vi "ProcessUDPValues.vi"(8 "error in (no error)":errorcluster, 11 "connection ID":refnum<k16>) -> ()   [LabVIEW 2015]
uses:
  GlobalVisionVars.vi
  navx-mxp/labview/navX Library v2/navX Library v2.lvlib
panel:
  out "ProcessTime":dbl
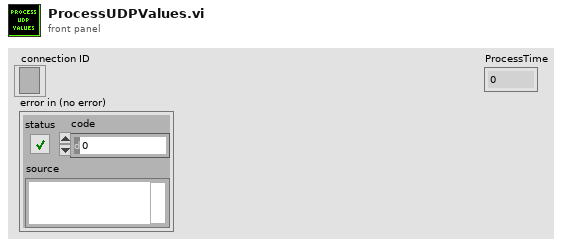
[diagram p1: front panel]
types:
  T1 = typedef "navX Library v2.lvlib/Z900_navX_DeviceTypeDef.ctl" = cluster{"Interface":cluster{"Protocol":T2, "Update Rate (4Hz-100Hz)":u8, "navX Open TypeDef":variant}, "Notify Packet":refnum<notifier>, "Loop VI Refnum":refnum<vi>, "Ready to Close Occurrence Refnum":refnum<k4>}
  T2 = typedef "navX Library v2.lvlib/Z900_navX_ProtocolTypeDef.ctl" = enum16{"SERIAL", "I2C", "SPI"}
  T3 = cluster{"Yaw":dbl, "Roll":dbl, "Pitch":dbl, "Heading":dbl, "Fused Heading":dbl}
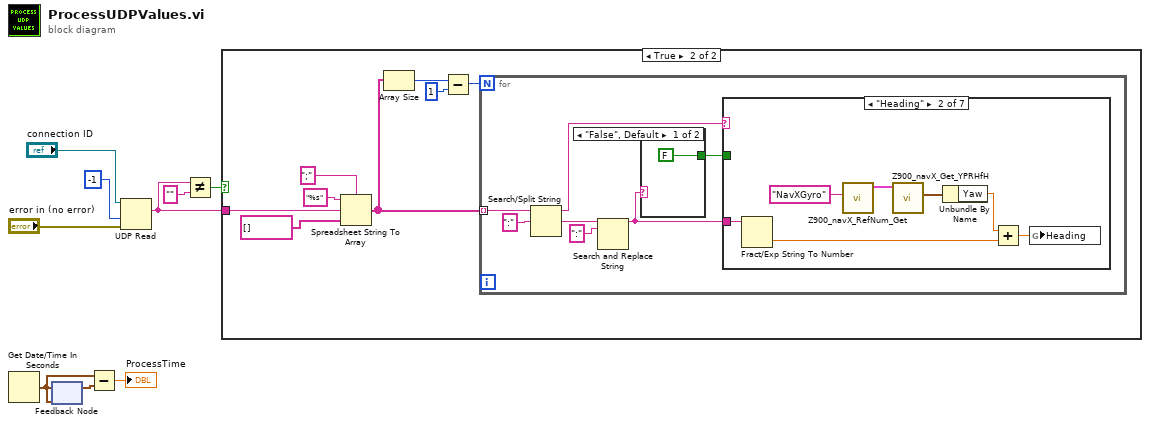
[diagram p0: block diagram]
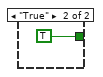
[diagram p3: hidden frame]
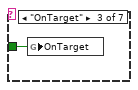
[diagram p5: hidden frame]
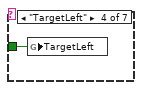
[diagram p6: hidden frame]
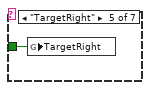
[diagram p7: hidden frame]
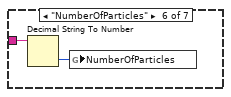
[diagram p8: hidden frame]
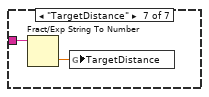
[diagram p9: hidden frame]
diagram:
  n1 = Get Date/Time In Seconds() -> (seconds since 1Jan1904=w7:timestamp)
  n2 = feedback-in #1(w7) -> ()
  n3 = feedback #1(w7) -> (w9:timestamp)
  n4 = Subtract(x=w7, y=w9) -> (x-y=→"ProcessTime":dbl)
  n5 = UDP Read(connection ID="connection ID", timeout ms (25000)=-1, 8:"error in (no error)") -> (data out=w1:string)  [unwired: 1 in, 4 out]
  n6 = Not Equal?(x=w1, y="") -> (x != y?=w2:bool)
  n7 = case shown="True" w2 {
    tunnel: w1 -> [_ w17]
    frame False {
    }
    frame True {
      n8 = Spreadsheet String To Array(delimiter (Tab)=";" ("search string/char (-)"), format string="%s", spreadsheet string=w17, array type (2D Dbl)=string[] []) -> (array=w13:string[])
      n9 = Array Size(array=w13) -> (size(s)=w12:i32)
      n10 = Subtract(x=w12, y=1) -> (x-y=w10:i32)
      n11 = for {
        N: w10 -> [_]
        tunnel: w13 -> [w24] mode=indexing
        n12 = Search/Split String(string=w24, search string/char (-)=":") -> (substring before match=w22:string, match + rest of string=w21:string)  [unwired: 1 in, 1 out]
        n13 = Search and Replace String(input string=w21, search string=":" ("replace string (\"\")")) -> (result string=w19:string)  [unwired: 6 in, 3 out]
        n14 = case shown="\"False\", Default" w19 {
          tunnel: [FALSE TRUE] -> w18
          frame "False", Default {
          }
          frame "True" {
          }
        }
        n15 = case shown="\"Heading\"" w22 {
          tunnel: w19 -> [_ w33 _ _ _ w38 w39]
          tunnel: w18 -> [_ _ w34 w35 w36 _ _]
          frame "False", Default {
          }
          frame "Heading" {
            n16 = Fract/Exp String To Number(string=w33) -> (number=w27:dbl)  [unwired: 3 in, 1 out]
            n17 = call "Z900_navX_RefNum_Get.vi"("refnum name"="NavXGyro") -> ("navX Device"=w32:T1)  [unwired: 9 in, 1 out]
            n18 = call "Z900_navX_Get_YPRHfH.vi"("navX Device"=w32) -> ("YRPHfH"=w31:T3)  [unwired: 7 in, 3 out]
            n19 = Unbundle By Name(w31) -> ("Yaw"=w29:dbl)
            n20 = Add(x=w29, y=w27) -> (x+y=w28:dbl)
            n21 = global write "GlobalVisionVars.vi" "Heading"(w28) -> ()
          }
          frame "OnTarget" {
            n22 = global write "GlobalVisionVars.vi" "OnTarget"(w34) -> ()
          }
          frame "TargetLeft" {
            n23 = global write "GlobalVisionVars.vi" "TargetLeft"(w35) -> ()
          }
          frame "TargetRight" {
            n24 = global write "GlobalVisionVars.vi" "TargetRight"(w36) -> ()
          }
          frame "NumberOfParticles" {
            n25 = Decimal String To Number(string=w38) -> (number=w37:i32)  [unwired: 2 in, 1 out]
            n26 = global write "GlobalVisionVars.vi" "NumberOfParticles"(w37) -> ()
          }
          frame "TargetDistance" {
            n27 = Fract/Exp String To Number(string=w39) -> (number=w40:dbl)  [unwired: 3 in, 1 out]
            n28 = global write "GlobalVisionVars.vi" "TargetDistance"(w40) -> ()
          }
        }
      }
    }
  }
